vi "PWM Read Frequency.vi"(7 "GPIO #":T1=-1, 8 "error in (no error)":errorcluster, 11 "VisaComms in":refnum<class "VisaComms.lvclass">) -> (0 "error out":errorcluster, 2 "Frequency Hz":sgl, 3 "VisaComms out":refnum<class "VisaComms.lvclass">)   [LabVIEW 2020, in "CTI.lvlib" / "VisaComms.lvclass"]
uses:
  VisaComms.lvclass
  GPIO Number.ctl
  VisaComms.lvclass/VisaComms.ctl
  CTI.lvlib
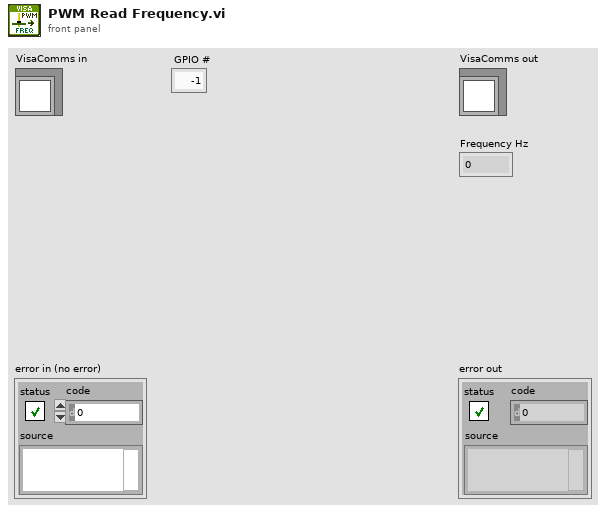
[diagram p1: front panel]
types:
  T1 = typedef "CTI.lvlib/GPIO Number.ctl" = i8
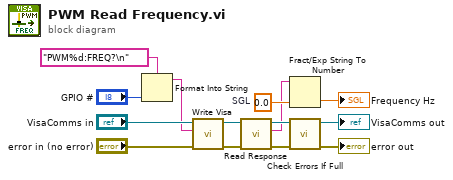
[diagram p0: block diagram]
diagram:
  w12 = sgl 0.0  # SGL
  n1 = Format Into String(format string="PWM%d:FREQ?\n", "GPIO #") -> (resulting string=w5:string)  [unwired: 2 in, 1 out]
  n2 = call "Write Visa.vi"("error in (no error)"="error in (no error)", "write buffer"=w5, "VisaComms in"="VisaComms in") -> ("error out"=w7:errorcluster, "VisaComms out"=w3:refnum<class "VisaComms.lvclass">)  [unwired: 6 in, 1 out]
  n3 = call "Read Response.vi"("error in (no error)"=w7, "VisaComms in"=w3) -> ("error out"=w4:errorcluster, "Response"=w1:string, "VisaComms out"=w2:refnum<class "VisaComms.lvclass">)  [unwired: 6 in, 1 out]
  n4 = Fract/Exp String To Number(string=w1, default (0 dbl)=w12) -> (number=→"Frequency Hz":sgl)  [unwired: 2 in, 1 out]
  n5 = call "Check Errors If Full.vi"("error in (no error)"=w4, "VisaComms in"=w2) -> ("error out"=→"error out":errorcluster, "VisaComms out"=→"VisaComms out":refnum<class "VisaComms.lvclass">)  [unwired: 8 in]
